vi "Motor-HandPaddle2D.vi"(0 "Motor Y":string, 1 "Motor X":string) -> ()   [LabVIEW 2009]
uses:
  Ressources/StopUserEvent.ctl
  Ressources/Stop.ctl
panel:
  in  "Up":bool
  in  "Left":bool
  in  "Right":bool
  in  "Down":bool
  out "Y":i32
  out "X":i32
  in  "Step Size":i32(slide) scale=0.0..100.0
  in  "stop":bool
  out "Stop User Event":T1
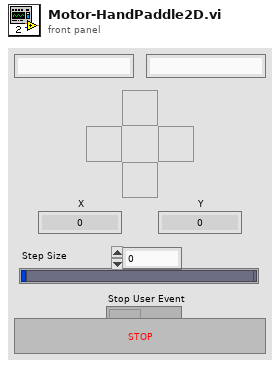
[diagram p1: front panel]
types:
  T1 = typedef "StopUserEvent.ctl" = refnum<user-event>
  T2 = typedef "Stop.ctl" = bool
  T3 = typedef "MotorStatus.ctl" = cluster{"Managed?":bool, "Position":i32, "Name":string, "Status":enum16{"OFF", "IDLE", "MOVING", "HOMING"}}
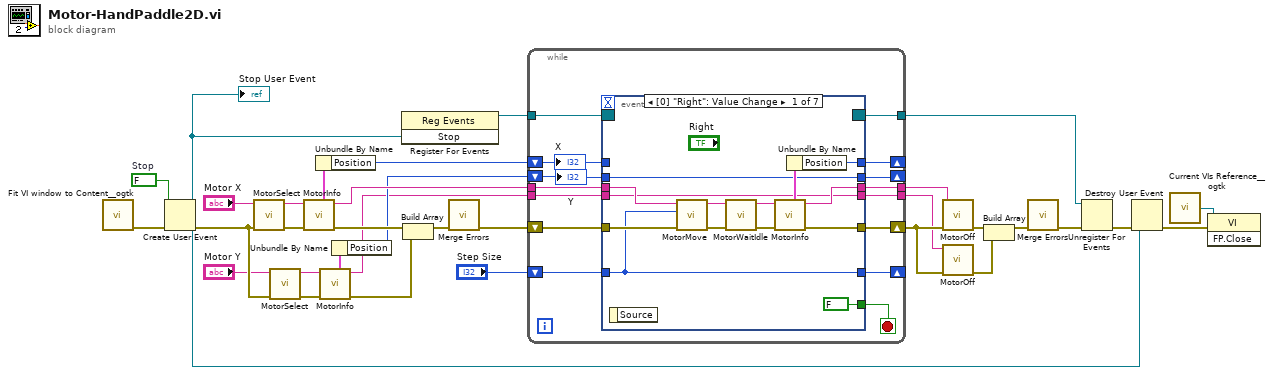
[diagram p0: block diagram]
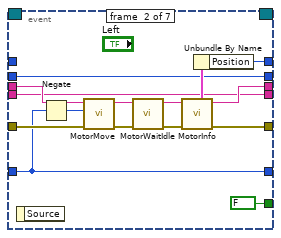
[diagram p2: hidden frame]
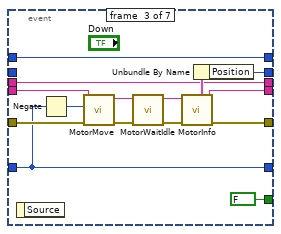
[diagram p3: hidden frame]
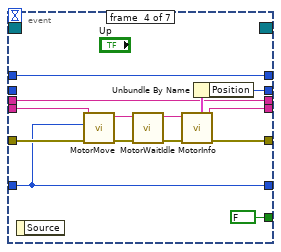
[diagram p4: hidden frame]
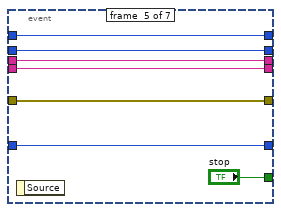
[diagram p5: hidden frame]
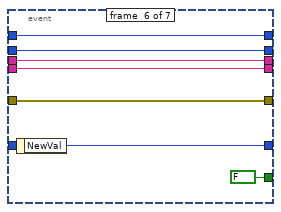
[diagram p6: hidden frame]
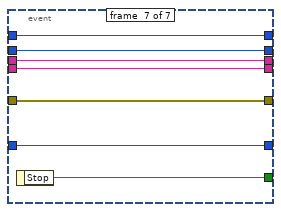
[diagram p7: hidden frame]
diagram:
  w20 = T2 FALSE  # Stop
  n1 = call <userlib>:"Fit VI window to Content__ogtk.vi"() -> ("error out"=w21:errorcluster)  [unwired: 3 in, 4 out]
  n2 = Create User Event(user event datatype=w20, error in=w21) -> (user event=w19:refnum<user-event>, error out=w15:errorcluster)
  "Stop User Event" <- w19
  n3 = call "MotorSelect.vi"("Motor"="Motor X", "error in (no error)"=w15) -> ("Motor out"=w30:string, "error out"=w31:errorcluster)  [unwired: 6 out]
  n4 = call "MotorSelect.vi"("Motor"="Motor Y", "error in (no error)"=w15) -> ("Motor out"=w17:string, "error out"=w16:errorcluster)  [unwired: 6 out]
  n5 = call "MotorInfo.vi"("error in (no error)"=w31, "Motor"=w30) -> ("error out"=w13:errorcluster, "Motor out"=w29:string, "Axis status"=w28:T3)  [unwired: 5 out]
  n6 = Unbundle By Name(w28) -> ("Position"=w27:i32)
  n7 = call "MotorInfo.vi"("error in (no error)"=w16, "Motor"=w17) -> ("error out"=w12:errorcluster, "Motor out"=w8:string, "Axis status"=w18:T3)  [unwired: 5 out]
  n8 = Unbundle By Name(w18) -> ("Position"=w11:i32)
  n9 = register-events(w19) -> (reference out=w26:refnum<event-registration>)  [unwired: 2 in, 1 out]
  n10 = Build Array(w13, w12) -> (w9:errorcluster[])
  n11 = call <vilib>:"Merge Errors.vi"("error array in"=w9) -> ("error out"=w10:errorcluster)  [unwired: 6 in]
  n12 = while {
    shift-right: [w46] -> w7
    shift-left: w10 -> [w48]
    tunnel: w29 -> [w47]
    tunnel: [w45] -> w4
    shift-right: [w43] -> _
    shift-left: "Step Size" -> [w44]
    shift-right: [w42] -> _
    shift-left: w27 -> [w41]
    tunnel: w26 -> [w39]
    tunnel: [w38] -> w25
    shift-right: [w35] -> _
    shift-left: w11 -> [w37]
    tunnel: w8 -> [w36]
    tunnel: [w34] -> w3
    stop <- w40 stop-if-true
    n13 = event shown="[0] \"Right\": Value Change" {
      selector: w39 -> [_ _ _ _ _ _ _]
      dyn-events: [_ _ _ _ _ _ _] -> w38
      timeout: _ -> [_ _ _ _ _ _ _]
      tunnel: w48 -> [w60 w75 w90 w104 w111 w118 w124]
      tunnel: w47 -> [w59 w74 w78 w94 w112 w119 w123]
      tunnel: [w54 w69 w85 w100 w111 w118 w124] -> w46
      tunnel: [w53 w68 w78 w94 w112 w119 w123] -> w45
      tunnel: w44 -> [w58 w73 w89 w95 w110 _ w125]
      tunnel: [w58 w73 w89 w95 w110 w120 w125] -> w43
      tunnel: [w52 w67 w80 w96 w113 w117 w126] -> w42
      tunnel: w41 -> [_ _ w80 w96 w113 w117 w126]
      tunnel: [FALSE ("stop") FALSE ("stop") FALSE ("stop") FALSE ("stop") "stop" FALSE ("stop") w127] -> w40
      tunnel: w37 -> [w50 w65 _ _ w108 w115 w122]
      tunnel: w36 -> [w49 w63 w82 w98 w107 w114 w121]
      tunnel: [w50 w65 w81 w97 w108 w115 w122] -> w35
      tunnel: [w49 w63 w79 w93 w107 w114 w121] -> w34
      event #0 {
        n14 = event-data() -> ()  [unwired: 2 out]
        n15 = call "MotorMove.vi"("Motor"=w59, "Movement"=w58, "error in (no error)"=w60) -> ("Motor out"=w61:string, "error out"=w62:errorcluster)  [unwired: 5 out]
        n16 = call "MotorWaitIdle.vi"("Motor"=w61, "error in (no error)"=w62) -> ("Motor out"=w56:string, "error out"=w55:errorcluster)  [unwired: 6 out]
        n17 = call "MotorInfo.vi"("error in (no error)"=w55, "Motor"=w56) -> ("error out"=w54:errorcluster, "Motor out"=w53:string, "Axis status"=w57:T3)  [unwired: 5 out]
        n18 = Unbundle By Name(w57) -> ("Position"=w52:i32)
      }
      event #1 {
        n19 = event-data() -> ()  [unwired: 2 out]
        n20 = Negate(x=w73) -> (-x=w64:i32)
        n21 = call "MotorMove.vi"("Motor"=w74, "Movement"=w64, "error in (no error)"=w75) -> ("Motor out"=w76:string, "error out"=w77:errorcluster)  [unwired: 5 out]
        n22 = call "MotorWaitIdle.vi"("Motor"=w76, "error in (no error)"=w77) -> ("Motor out"=w71:string, "error out"=w70:errorcluster)  [unwired: 6 out]
        n23 = call "MotorInfo.vi"("error in (no error)"=w70, "Motor"=w71) -> ("error out"=w69:errorcluster, "Motor out"=w68:string, "Axis status"=w72:T3)  [unwired: 5 out]
        n24 = Unbundle By Name(w72) -> ("Position"=w67:i32)
      }
      event #2 {
        n25 = event-data() -> ()  [unwired: 2 out]
        n26 = Negate(x=w89) -> (-x=w83:i32)
        n27 = call "MotorMove.vi"("Motor"=w82, "Movement"=w83, "error in (no error)"=w90) -> ("Motor out"=w91:string, "error out"=w92:errorcluster)  [unwired: 5 out]
        n28 = call "MotorWaitIdle.vi"("Motor"=w91, "error in (no error)"=w92) -> ("Motor out"=w87:string, "error out"=w86:errorcluster)  [unwired: 6 out]
        n29 = call "MotorInfo.vi"("error in (no error)"=w86, "Motor"=w87) -> ("error out"=w85:errorcluster, "Motor out"=w79:string, "Axis status"=w88:T3)  [unwired: 5 out]
        n30 = Unbundle By Name(w88) -> ("Position"=w81:i32)
      }
      event #3 {
        n31 = event-data() -> ()  [unwired: 2 out]
        n32 = call "MotorMove.vi"("Motor"=w98, "Movement"=w95, "error in (no error)"=w104) -> ("Motor out"=w105:string, "error out"=w106:errorcluster)  [unwired: 5 out]
        n33 = call "MotorWaitIdle.vi"("Motor"=w105, "error in (no error)"=w106) -> ("Motor out"=w102:string, "error out"=w101:errorcluster)  [unwired: 6 out]
        n34 = call "MotorInfo.vi"("error in (no error)"=w101, "Motor"=w102) -> ("error out"=w100:errorcluster, "Motor out"=w93:string, "Axis status"=w103:T3)  [unwired: 5 out]
        n35 = Unbundle By Name(w103) -> ("Position"=w97:i32)
      }
      event #4 {
        n36 = event-data() -> ()  [unwired: 2 out]
      }
      event #5 {
        n37 = event-data() -> ("NewVal"=w120:i32)  [unwired: 1 out]
      }
      event #6 {
        n38 = event-data() -> ("Stop"=w127:T2)  [unwired: 1 out]
      }
    }
    "X" <- w41
    "Y" <- w37
  }
  n39 = call "MotorOff.vi"("Motor"=w4, "error in (no error)"=w7) -> ("error out"=w6:errorcluster)  [unwired: 7 out]
  n40 = call "MotorOff.vi"("Motor"=w3, "error in (no error)"=w7) -> ("error out"=w5:errorcluster)  [unwired: 7 out]
  n41 = Build Array(w6, w5) -> (w2:errorcluster[])
  n42 = call <vilib>:"Merge Errors.vi"("error array in"=w2) -> ("error out"=w1:errorcluster)  [unwired: 6 in]
  n43 = Unregister For Events(event registration refnum=w25, error in=w1) -> (error out=w24:errorcluster)
  n44 = Destroy User Event(user event=w19, error in=w24) -> (error out=w23:errorcluster)
  n45 = call <userlib>:"Current VIs Reference__ogtk.vi"() -> ("Current VI's reference"=w22:refnum<vi>)  [unwired: 5 out]
  n46 = invoke class="VI" method="FP.Close"(reference=w22, error in=w23) -> ()  [unwired: 1 in, 3 out]
